vi "Slide Servo home.vi"(8 "error in":errorcluster, 10 "NewVal":bool) -> (0 "error out":errorcluster)   [LabVIEW 2015]
uses:
  Project Setup/Globle Variable/GR_Servo.vi
  Galobal variable_TI.vi
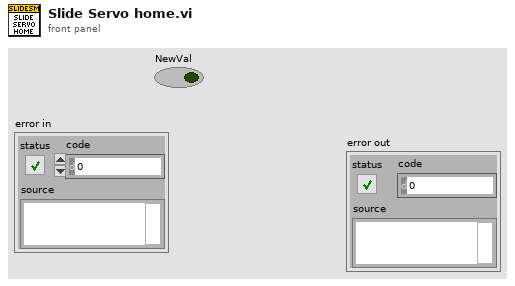
[diagram p1: front panel]
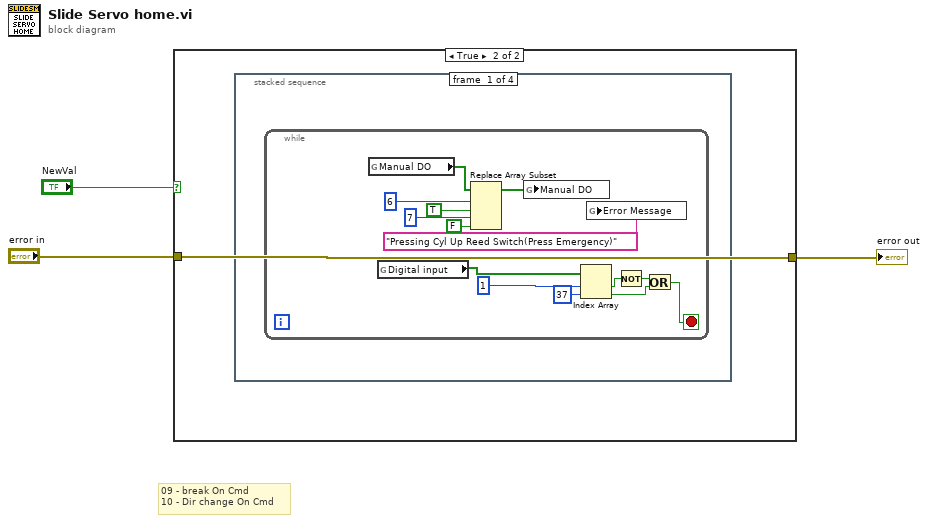
[diagram p0: block diagram]
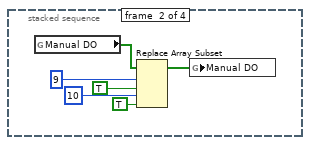
[diagram p3: hidden frame]
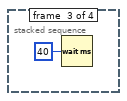
[diagram p4: hidden frame]
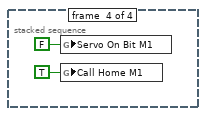
[diagram p5: hidden frame]
diagram:
  # "09 - break On Cmd\n10 - Dir change On Cmd"
  n1 = case shown="True" "NewVal" {
    tunnel: "error in" -> [w4 w5]
    tunnel: [w4 w5] -> w1
    frame False {
    }
    frame True {
      n2 = stacked-sequence {
        frame #0 {
          n3 = while {
            stop <- w7 stop-if-true
            n4 = global read "Galobal variable_TI.vi" "Manual DO"() -> (w15:bool[])
            n5 = global read "Galobal variable_TI.vi" "Digital input"() -> (w13:bool[])
            n6 = Replace Array Subset(array=w15, new element #1=TRUE ("new element/subarray"), index #1=6 ("index"), new element #2=FALSE ("new element/subarray"), index #2=7 ("index")) -> (w19:bool[])
            n7 = global write "Galobal variable_TI.vi" "Manual DO"(w19) -> ()
            n8 = Index Array(array=w13, index #1=1 ("index"), index #2=37 ("index")) -> (element #1=w11:bool, element #2=w8:bool)
            n9 = global write "GR_Servo.vi" "Error Message"("Pressing Cyl Up Reed Switch(Press Emergency)") -> ()
            n10 = Not(x=w11) -> (.not. x?=w10:bool)
            n11 = Or(x=w10, y=w8) -> (x .or. y?=w7:bool)
          }
        }
        frame #1 {
          n12 = global read "Galobal variable_TI.vi" "Manual DO"() -> (w21:bool[])
          n13 = Replace Array Subset(array=w21, new element #1=TRUE ("new element/subarray"), index #1=9 ("index"), new element #2=TRUE ("new element/subarray"), index #2=10 ("index")) -> (w25:bool[])
          n14 = global write "Galobal variable_TI.vi" "Manual DO"(w25) -> ()
        }
        frame #2 {
          n15 = Wait (ms)(milliseconds to wait=u32 40) -> ()  [unwired: 1 out]
        }
        frame #3 {
          n16 = global write "GR_Servo.vi" "Servo On Bit M1"(FALSE ("Servo On Bit")) -> ()
          n17 = global write "Galobal variable_TI.vi" "Call Home M1"(TRUE ("Call Home M1")) -> ()
        }
      }
    }
  }
  "error out" <- w1
